vi "Fetch - NT Scalar (Numeric).vi"(7 "PV name":string, 8 "error in":errorcluster, 10 "default value":refnum<class "NT Scalar (Numeric).lvclass">, 11 "Server in":refnum<class "Server.lvclass">) -> (0 "error out":errorcluster, 1 "PV not found?":bool, 2 "value":refnum<class "NT Scalar (Numeric).lvclass">, 3 "Server out":refnum<class "Server.lvclass">)   [LabVIEW 2020, in "PV Access.lvlib" / "PVA Server.lvlib" / "Server.lvclass"]
uses:
  Server.lvclass
  Server.lvclass/Server.ctl
  2889940d-94b1-4eb8-afd7-6f859beffe7f.vi
  PV Data/NT Scalar (Numeric)/NT Scalar (Numeric).lvclass
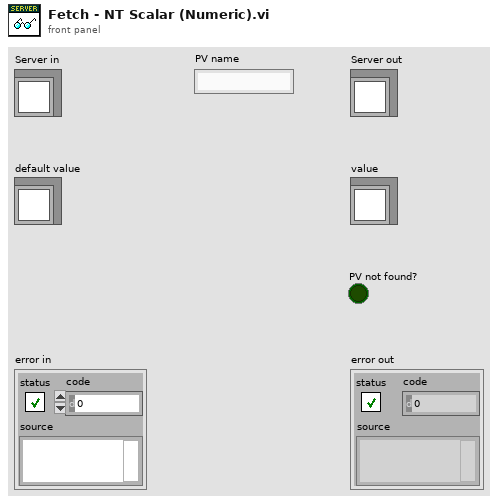
[diagram p1: front panel]
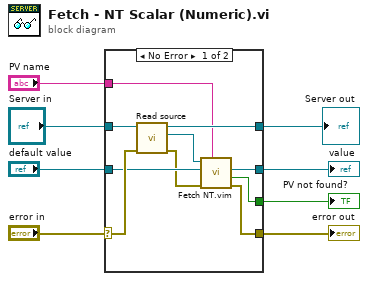
[diagram p0: block diagram]
diagram:
  n1 = case shown="No Error" "error in" {
    selector: "error in" -> [w18 w19]
    tunnel: [w11 w19] -> w7
    tunnel: "PV name" -> [w14 _]
    tunnel: "Server in" -> [w17 w21]
    tunnel: [w16 w21] -> w4
    tunnel: "default value" -> [w13 w20]
    tunnel: [w12 w20] -> w5
    tunnel: [w9 _] -> w6
    frame No Error {
      n2 = call "Read source.vi"("error in (no error)"=w18, "Server in"=w17) -> ("error out"=w10:errorcluster, "Source"=w15:refnum<class "Source.lvclass">, "Server out"=w16:refnum<class "Server.lvclass">)  [unwired: 7 in]
      n3 = call "Fetch NT.vim"("PV name"=w14, "error in"=w10, "default value"=w13, "Source in"=w15) -> ("error out"=w11:errorcluster, "PV not found?"=w9:bool, "value"=w12:refnum<class "NT Scalar (Numeric).lvclass">)  [unwired: 4 in, 1 out]
    }
    frame Error {
    }
  }
  "Server out" <- w4
  "error out" <- w7
  "value" <- w5
  "PV not found?" <- w6
